vi "EncoderInit.vi"(0 "refnum name":string="LDriveEncoder", 1 "DistancePerCount":dbl=0.02399827721492203, 2 "DIO Channel":T1, 3 "DIO Channel 2":T1) -> ()   [LabVIEW 2012]
uses:
  <vilib>/Rock Robotics/SystemInterfaces/DIO/FPGA_DIOChannel.ctl
  <vilib>/Rock Robotics/WPI/Encoder/WPI_EncoderType.ctl
  <vilib>/Rock Robotics/WPI/Counter/WPI_CounterDigitalInputToDigitalSource.vi
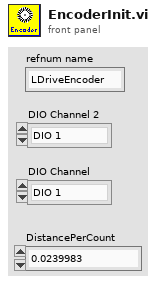
[diagram p1: front panel]
types:
  T1 = typedef "FPGA_DIOChannel.ctl" = enum8{"DIO 1", "DIO 2", "DIO 3", "DIO 4", "DIO 5", "DIO 6", "DIO 7", "DIO 8", "DIO 9", "DIO 10", "DIO 11", "DIO 12", "DIO 13", "DIO 14", "Invalid"}
  T2 = typedef "WPI_EncoderType.ctl" = enum16{"1x", "2x", "4x"}
  T3 = typedef "WPI_DigitalInputDevRef.ctl" = cluster{"DevStatus":errorcluster, "DIO Channel":T1, "Digital Module":T4}
  T4 = typedef "FPGA_TypedefDigitalModule.ctl" = enum16{"Digital Module 1", "Digital Module 2"}
  T5 = typedef "FPGA_CounterEncoderSourceConvertionLVSourceType.ctl" = cluster{"DevStatus":errorcluster, "AnalogTriggerMode?":bool, "DigitalMode":cluster{"Digital Module":T4, "DIO Channel":T6}, "AnalogTriggerMode":cluster{"AnalogTriggerIndex":T7, "OutputType":T8}}
  T6 = typedef "FPGA_DIODigitalSourceChannel.ctl" = enum8{"DIO 1", "DIO 2", "DIO 3", "DIO 4", "DIO 5", "DIO 6", "DIO 7", "DIO 8", "DIO 9", "DIO 10", "DIO 11", "DIO 12", "DIO 13", "DIO 14", "Disabled"}
  T7 = typedef "FPGA_AnalogTriggerIndex.ctl" = enum8{"Trig 0", "Trig 1", "Trig 2", "Trig 3", "Trig 4", "Trig 5", "Trig 6", "Trig 7", "Invalid"}
  T8 = typedef "FPGA_AnalogTriggerOutType.ctl" = enum16{"InWindow", "TriggerState", "Rising", "Falling"}
  T9 = typedef "WPI_EncoderDevRef.ctl" = cluster{"DevStatus":errorcluster, "EncoderIndex":T10, "CounterIndex":T11, "DistancePerCount":dbl, "Decoding Type":T2}
  T10 = typedef "FPGA_EncoderIdx.ctl" = enum8{"Enc 0", "Enc 1", "Enc 2", "Enc 3", "Invalid"}
  T11 = typedef "FPGA_CounterCtrSystemIndex.ctl" = enum8{"Ctr 0", "Ctr 1", "Ctr 2", "Ctr 3", "Ctr 4", "Ctr 5", "Ctr 6", "Ctr 7", "Invalid"}
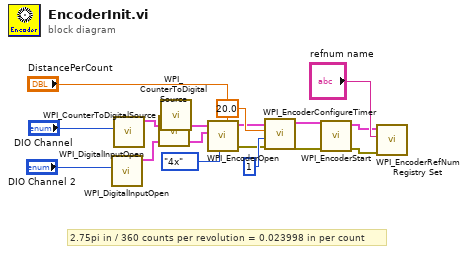
[diagram p0: block diagram]
diagram:
  # "2.75pi in / 360 counts per revolution = 0.023998 in per count"
  n1 = call <vilib>:"WPI_DigitalInputOpen.vi"("DIO Channel"="DIO Channel 2") -> ("DigitalInputDevRef"=w6:T3)  [unwired: 9 in, 1 out]
  n2 = call <vilib>:"WPI_DigitalInputOpen.vi"("DIO Channel"="DIO Channel") -> ("DigitalInputDevRef"=w9:T3)  [unwired: 9 in, 1 out]
  n3 = call-poly <vilib>:"WPI_CounterToDigitalSource.vi"("DigitalInputDevRef"=w6) -> ("Digital Source"=w5:T5)  [unwired: 6 in]
  n4 = call-poly <vilib>:"WPI_CounterToDigitalSource.vi"("DigitalInputDevRef"=w9) -> ("Digital Source"=w10:T5)  [unwired: 6 in]
  n5 = call <vilib>:"WPI_EncoderOpen.vi"("DistancePerCount"="DistancePerCount", "Decoding Type"=WPI_EncoderType."4x", "BSource"=w5, "ASource"=w10) -> ("error out"=w15:errorcluster, "EncoderDevRef"=w12:T9)  [unwired: 6 in]
  n6 = call <vilib>:"WPI_EncoderConfigureTimer.vi"("error in (no error)"=w15, "Number Samples to Average"=u8 1, "Minimum Rate"=20.0, "EncoderDevRef"=w12) -> ("error out"=w14:errorcluster, "EncoderDevRef"=w13:T9)  [unwired: 6 in]
  n7 = call <vilib>:"WPI_EncoderStart.vi"("error in (no error)"=w14, "EncoderDevRef"=w13) -> ("error out"=w2:errorcluster, "EncoderDevRef"=w3:T9)  [unwired: 8 in]
  n8 = call <vilib>:"WPI_EncoderRefNum Registry Set.vi"("error in (no error)"=w2, "refnum name"="refnum name", "EncoderDevRef"=w3) -> ()  [unwired: 7 in, 2 out]
